vi "Axes Deadband.vi"(10 "limit":dbl, 11 "valueIn":dbl) -> (0 "inDeadband":bool, 3 "valueOut":dbl)   [LabVIEW 2019]
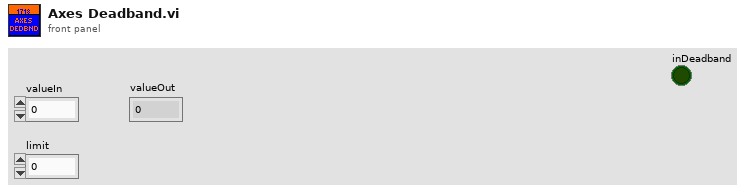
[diagram p1: front panel]
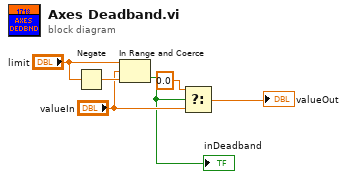
[diagram p0: block diagram]
diagram:
  n1 = Negate(x="limit") -> (-x=w5:dbl)
  n2 = In Range and Coerce(upper limit="limit", x="valueIn", lower limit=w5) -> (In Range?=w1:bool)  [unwired: 1 out]
  "inDeadband" <- w1
  n3 = Select(t=0.0, s=w1, f="valueIn") -> (s? t:f=→"valueOut":dbl)
